vi "Configure Digital Filter.vi"(0 "VISA resource name":refnum<visa-resource-name>, 1 "Measurement (0: Voltage Channel 1)":i32(ring) items=["Voltage Channel 1", "Voltage Channel 2", "Temperature Channel 1", "Temperature Channel 2"], 5 "Enable Digital Filter (T: Enable)":bool=TRUE, 7 "Filter Window (0.01%)":dbl=0.01, 9 "Filter Count (10)":i32=10, 11 "error in (no error)":errorcluster, 12 "Filter Type (0: Moving)":i32(ring) items=["Moving", "Repeat"]) -> (4 "VISA resource name out":refnum<visa-resource-name>, 15 "error out":errorcluster)   [LabVIEW 2021, in "Keithley 2182.lvlib"]
doc: "Configures the specified measurement's digital filter.\n\nThe digital filter is used to stabilize noisy measurements. The displayed, stored or transmitted reading is a windowed-average of a number of reading conversions (from 1 to 100).\n\nIn general, the digital filter places a specified number of A/D conversions (Filter Count) into a memory stack. These A/D conversions must occur consecutively within a selected reading window (Filter Window). The readings in the stack are then averaged to yield a single filtered reading. The stack can be filled in two ways (Filter Type); moving or repeating. The moving filter keeps adding and removing a single A/D conversion from the stack before taking the average, while the repeating filter only averages a stack that is filled with new A/D conversions.\n\n<B>Note:</B>\nWhen performing Ratio calculations, configured filter for V1 is automatically applied to V2."
uses:
  <instrlib>/Keithley 2182/Keithley 2182.lvlib
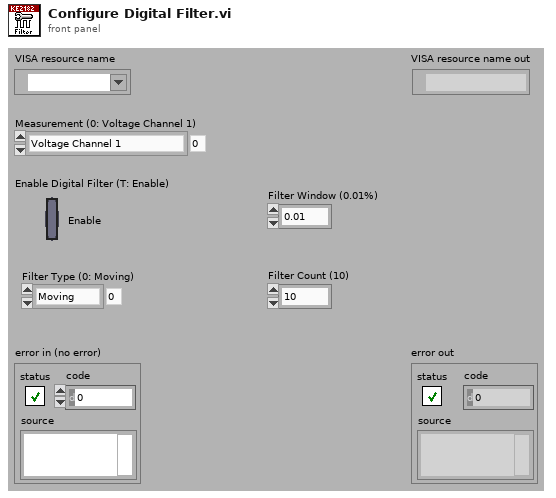
[diagram p1: front panel]
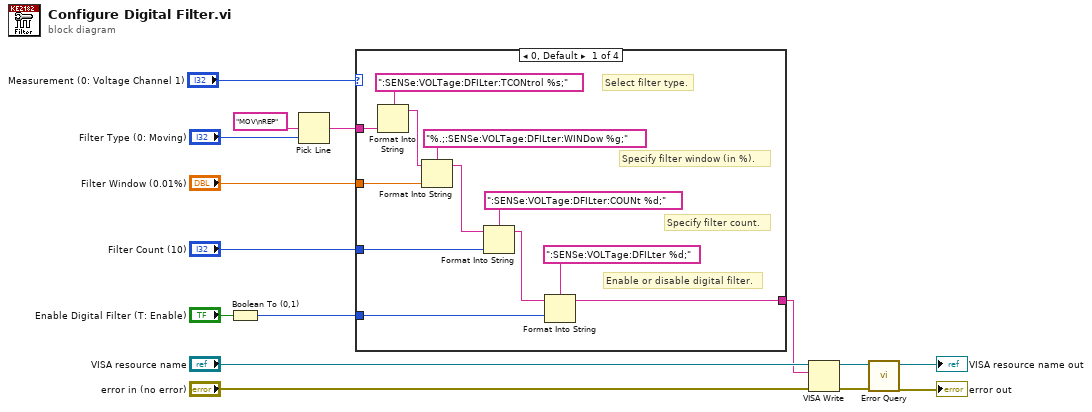
[diagram p0: block diagram]
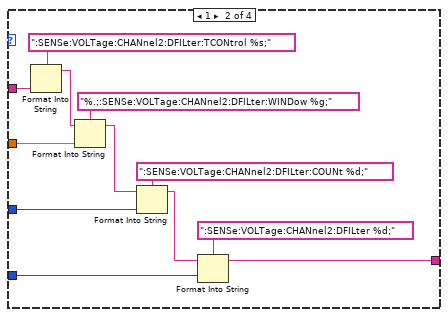
[diagram p2: hidden frame]
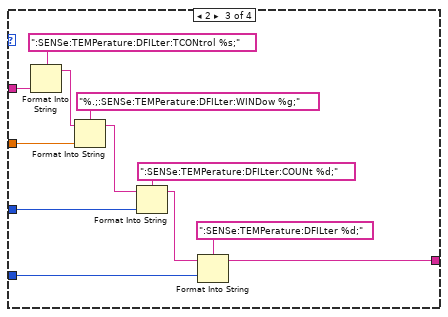
[diagram p3: hidden frame]
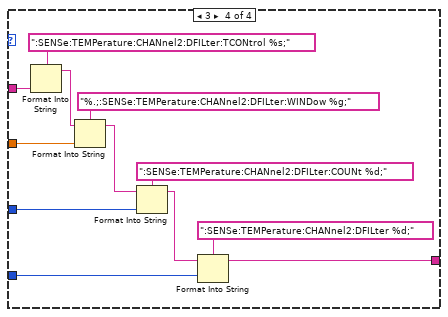
[diagram p4: hidden frame]
diagram:
  n1 = Boolean To (0,1)(Boolean="Enable Digital Filter (T: Enable)") -> (0, 1=w7:i16)
  n2 = Pick Line(multi-line string="MOV\nREP", line index="Filter Type (0: Moving)") -> (output string=w3:string)  [unwired: 1 in]
  n3 = case shown="0, Default" "Measurement (0: Voltage Channel 1)" {
    tunnel: w7 -> [w26 w38 w50 w62]
    tunnel: "Filter Count (10)" -> [w24 w36 w48 w60]
    tunnel: "Filter Window (0.01%)" -> [w21 w33 w45 w57]
    tunnel: w3 -> [w19 w31 w43 w55]
    tunnel: [w16 w28 w40 w52] -> w1
    frame 0, Default {
      # "Specify filter count."
      # "Enable or disable digital filter."
      # "Specify filter window (in %)."
      # "Select filter type."
      n4 = Format Into String(format string=":SENSe:VOLTage:DFILter:TCONtrol %s;", w19) -> (resulting string=w20:string)  [unwired: 2 in, 1 out]
      n5 = Format Into String(format string="%.;:SENSe:VOLTage:DFILter:WINDow %g;", initial string=w20, w21) -> (resulting string=w22:string)  [unwired: 1 in, 1 out]
      n6 = Format Into String(format string=":SENSe:VOLTage:DFILter:COUNt %d;", initial string=w22, w24) -> (resulting string=w23:string)  [unwired: 1 in, 1 out]
      n7 = Format Into String(format string=":SENSe:VOLTage:DFILter %d;", initial string=w23, w26) -> (resulting string=w16:string)  [unwired: 1 in, 1 out]
    }
    frame 1 {
      n8 = Format Into String(format string=":SENSe:VOLTage:CHANnel2:DFILter:TCONtrol %s;", w31) -> (resulting string=w32:string)  [unwired: 2 in, 1 out]
      n9 = Format Into String(format string="%.;:SENSe:VOLTage:CHANnel2:DFILter:WINDow %g;", initial string=w32, w33) -> (resulting string=w34:string)  [unwired: 1 in, 1 out]
      n10 = Format Into String(format string=":SENSe:VOLTage:CHANnel2:DFILter:COUNt %d;", initial string=w34, w36) -> (resulting string=w35:string)  [unwired: 1 in, 1 out]
      n11 = Format Into String(format string=":SENSe:VOLTage:CHANnel2:DFILter %d;", initial string=w35, w38) -> (resulting string=w28:string)  [unwired: 1 in, 1 out]
    }
    frame 2 {
      n12 = Format Into String(format string=":SENSe:TEMPerature:DFILter:TCONtrol %s;", w43) -> (resulting string=w44:string)  [unwired: 2 in, 1 out]
      n13 = Format Into String(format string="%.;:SENSe:TEMPerature:DFILter:WINDow %g;", initial string=w44, w45) -> (resulting string=w46:string)  [unwired: 1 in, 1 out]
      n14 = Format Into String(format string=":SENSe:TEMPerature:DFILter:COUNt %d;", initial string=w46, w48) -> (resulting string=w47:string)  [unwired: 1 in, 1 out]
      n15 = Format Into String(format string=":SENSe:TEMPerature:DFILter %d;", initial string=w47, w50) -> (resulting string=w40:string)  [unwired: 1 in, 1 out]
    }
    frame 3 {
      n16 = Format Into String(format string=":SENSe:TEMPerature:CHANnel2:DFILter:TCONtrol %s;", w55) -> (resulting string=w56:string)  [unwired: 2 in, 1 out]
      n17 = Format Into String(format string="%.;:SENSe:TEMPerature:CHANnel2:DFILter:WINDow %g;", initial string=w56, w57) -> (resulting string=w58:string)  [unwired: 1 in, 1 out]
      n18 = Format Into String(format string=":SENSe:TEMPerature:CHANnel2:DFILter:COUNt %d;", initial string=w58, w60) -> (resulting string=w59:string)  [unwired: 1 in, 1 out]
      n19 = Format Into String(format string=":SENSe:TEMPerature:CHANnel2:DFILter %d;", initial string=w59, w62) -> (resulting string=w52:string)  [unwired: 1 in, 1 out]
    }
  }
  n20 = VISA Write(VISA resource name="VISA resource name", write buffer=w1, error in (no error)="error in (no error)") -> (VISA resource name out=w13:refnum<visa-resource-name>, error out=w12:errorcluster)  [unwired: 1 out]
  n21 = call <instrlib>:"Error Query.vi"("error in (no error)"=w12, "VISA resource name"=w13) -> ("error out"=→"error out":errorcluster, "VISA resource name out"=→"VISA resource name out":refnum<visa-resource-name>)  [unwired: 6 in, 2 out]
